vi "isConnected.vi"(8 "error in (no error)":errorcluster, 11 "Connection in":refnum<class "Connection.lvclass">) -> (0 "error out":errorcluster, 2 "connected":bool, 3 "Connection out":refnum<class "Connection.lvclass">)   [LabVIEW 2013, in "Connection_GOSPL.lvlib" / "Connection.lvclass"]
uses:
  Connection.lvclass
  Connection.lvclass/Connection.ctl
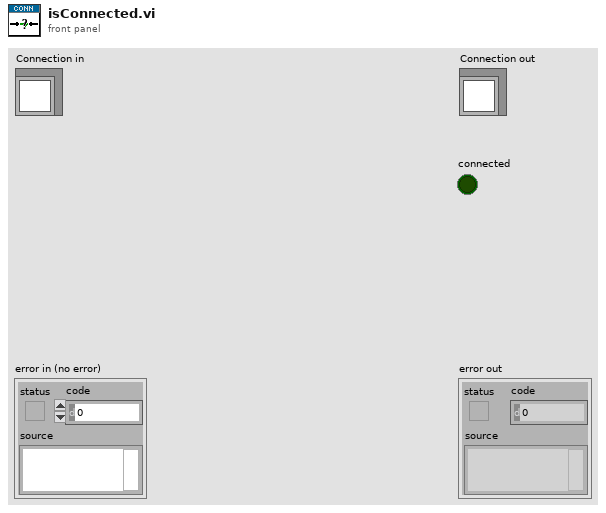
[diagram p1: front panel]
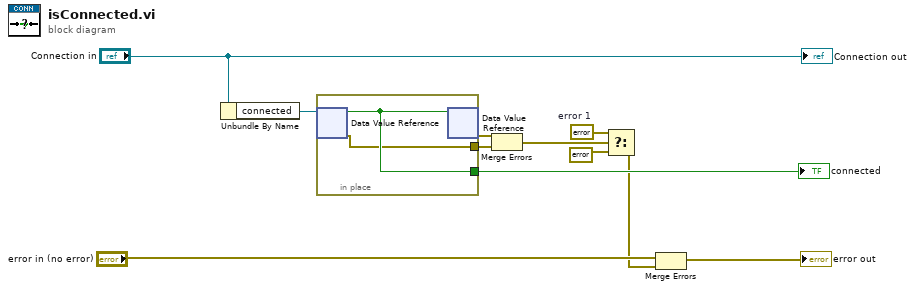
[diagram p0: block diagram]
diagram:
  w1 = errorcluster {"status"=TRUE, "code"=1, "source"="Connection_GOSPL.lvlib:Connection.lvclass:isConnected.vi"}  # error 1
  n1 = Unbundle By Name("Connection in") -> ("connected"=w10:refnum<data-value>)
  n2 = in-place {
    in-place-border: [w13] -> w9
    in-place-border: [w12] -> w6
    n3 = in-place-dvr #1(w10) -> (w13:bool, w12:errorcluster)
    n4 = in-place-dvr #1(w13) -> (w5:errorcluster)  [unwired: 1 out]
  }
  "connected" <- w9
  n5 = Merge Errors(w5, w6) -> (w4:errorcluster)
  n6 = Select(t=w1, s=w4, f=errorcluster {"status"=FALSE, "code"=0, "source"=""} ("error out")) -> (s? t:f=w2:errorcluster)
  n7 = Merge Errors("error in (no error)", w2) -> (→"error out":errorcluster)
  "Connection out" <- "Connection in"
